vi "DataLogging.vi"(4 "Tab?":bool, 6 "New Line?":bool, 7 "Name":string, 8 "error in (no error)":errorcluster, 10 "WriteToFile?":bool, 11 "Variant In":variant) -> (0 "error out":errorcluster, 3 "FinalText":string)   [LabVIEW 2017]
uses:
  <vilib>/Utility/Data Type/Type Definitions/Data Type.ctl
  <vilib>/Utility/Data Type/NI_Data Type.lvlib
panel:
  out "Type":T1
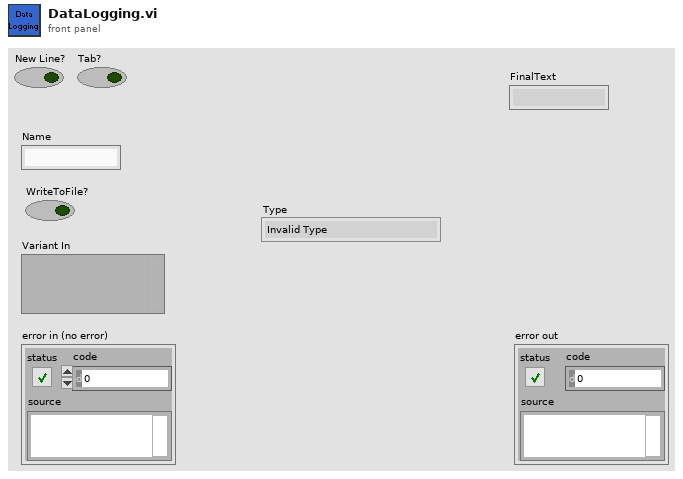
[diagram p1: front panel]
types:
  T1 = typedef "NI_Data Type.lvlib/Data Type.ctl" = enum8{"Invalid Type", "Void", "I8", "I16", "I32", "I64", "U8", "U16", "U32", "U64", "Single Float", "Double Float", "Extended Float", "Single Complex", "Double Complex", "Extended Complex", "Enum U8", "Enum U16", "Enum U32", "Enum U64", "Single Float With Unit", "Double Float With Unit", "Extended Float With Unit", "Single Complex with Unit", "Double Complex with Unit", "Extended Complex with Unit", "Boolean", "String", "Path", "Picture", "Tag", "Array", "Cluster", "Variant", "LV Variant", "Waveform", "Timestamp", "Digital Waveform", "Digital Data", "ExpressData", "Refnum", "External Data", "VI", "Poly VI", "LabVIEW Class Instance", "Fixed Point"}
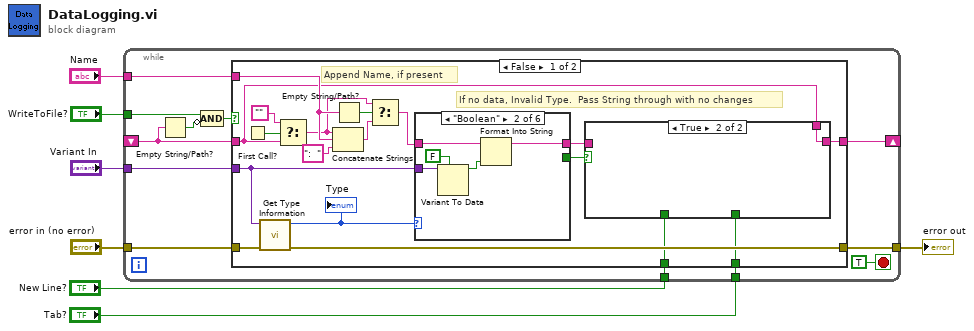
[diagram p0: block diagram]
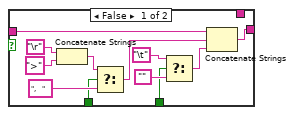
[diagram p2: hidden frame]
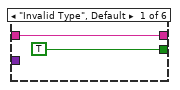
[diagram p3: hidden frame]
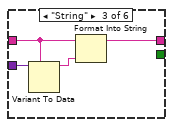
[diagram p4: hidden frame]
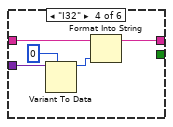
[diagram p5: hidden frame]
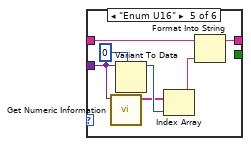
[diagram p6: hidden frame]
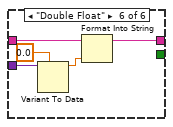
[diagram p7: hidden frame]
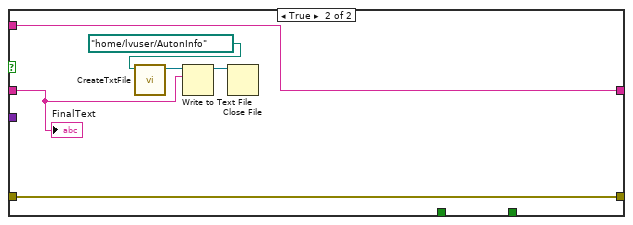
[diagram p8: hidden frame]
diagram:
  n1 = while {
    tunnel: "Variant In" -> [w19]
    shift-right: [w13] -> _
    shift-left: _ -> [w11]
    tunnel: "WriteToFile?" -> [w9]
    tunnel: "error in (no error)" -> [w17]
    tunnel: [w16] -> w4
    tunnel: "Name" -> [w15]
    tunnel: "New Line?" -> [w14]
    tunnel: "Tab?" -> [w12]
    stop <- TRUE stop-if-true
    n2 = Empty String/Path?(string/path=w11) -> (empty?=w8:bool)
    n3 = Compound Arithmetic op=AND(w9, invert w8) -> (w10:bool)
    n4 = case shown="False" w10 {
      tunnel: w19 -> [w37 _]
      tunnel: w17 -> [w36 w84]
      tunnel: [w35 w84] -> w16
      tunnel: w11 -> [w20 w80]
      tunnel: w15 -> [w31 w83]
      tunnel: w14 -> [w26 _]
      tunnel: [w21 w83] -> w13
      tunnel: w12 -> [w24 _]
      frame False {
        # "If no data, Invalid Type.  Pass String through with no changes"
        # "Append Name, if present"
        n5 = First Call?() -> (First Call?: T/F=w33:bool)
        n6 = call <vilib>:"Get Type Information.vi"("error in (no error)"=w36, "Variant"=w37) -> ("error out"=w35:errorcluster, "Type"=w23:T1)  [unwired: 5 in, 3 out]
        "Type" <- w23
        n7 = Select(t="", s=w33, f=w20) -> (s? t:f=w28:string)
        n8 = Concatenate Strings(w28, w31, ":  " ("string")) -> (w29:string)
        n9 = Empty String/Path?(string/path=w31) -> (empty?=w32:bool)
        n10 = Select(t=w28, s=w32, f=w29) -> (s? t:f=w30:string)
        n11 = case shown="\"Boolean\"" w23 {
          tunnel: w37 -> [_ w57 w61 w66 w69 w76]
          tunnel: [w52 w54 w59 w64 w73 w78] -> w25
          tunnel: w30 -> [w52 w53 w58 w63 w72 w77]
          tunnel: [TRUE _ _ _ _ _] -> w22
          frame "Invalid Type", Default {
          }
          frame "Boolean" {
            n12 = Variant To Data(type=FALSE, Variant=w57) -> (data=w55:bool)  [unwired: 1 in, 1 out]
            n13 = Format Into String(initial string=w53, w55) -> (resulting string=w54:string)  [unwired: 2 in, 1 out]
          }
          frame "String" {
            n14 = Variant To Data(type=w58, Variant=w61) -> (data=w60:string)  [unwired: 1 in, 1 out]
            n15 = Format Into String(initial string=w58, w60) -> (resulting string=w59:string)  [unwired: 2 in, 1 out]
          }
          frame "I32" {
            n16 = Variant To Data(type=0, Variant=w66) -> (data=w65:i32)  [unwired: 1 in, 1 out]
            n17 = Format Into String(initial string=w63, w65) -> (resulting string=w64:string)  [unwired: 2 in, 1 out]
          }
          frame "Enum U16" {
            n18 = call <vilib>:"Get Numeric Information.vi"("Variant"=w69) -> ("Enum Names"=w70:string[])  [unwired: 7 in, 3 out]
            n19 = Variant To Data(type=0, Variant=w69) -> (data=w71:i32)  [unwired: 1 in, 1 out]
            n20 = Index Array(array=w70, index=w71) -> (element=w68:string)
            n21 = Format Into String(initial string=w72, w68) -> (resulting string=w73:string)  [unwired: 2 in, 1 out]
          }
          frame "Double Float" {
            n22 = Variant To Data(type=0.0, Variant=w76) -> (data=w74:dbl)  [unwired: 1 in, 1 out]
            n23 = Format Into String(initial string=w77, w74) -> (resulting string=w78:string)  [unwired: 2 in, 1 out]
          }
        }
        n24 = case shown="True" w22 {
          tunnel: w26 -> [w46 _]
          tunnel: w25 -> [w45 _]
          tunnel: w24 -> [w39 _]
          tunnel: [w38 w50] -> w21
          tunnel: w20 -> [_ w50]
          frame False {
            n25 = Concatenate Strings("\r", ">") -> (w47:string)
            n26 = Select(t=w47, s=w46, f=",   ") -> (s? t:f=w44:string)
            n27 = Select(t="\t", s=w39, f="") -> (s? t:f=w42:string)
            n28 = Concatenate Strings(w45, w44, w42) -> (w38:string)
          }
          frame True {
          }
        }
      }
      frame True {
        n29 = call "CreateTxtFile.vi"("pathIn"=path "/home/lvuser/AutonInfo") -> ("refnumOut"=w81:refnum<file>)  [unwired: 10 in]
        n30 = Write to Text File(file (use dialog)=w81, text=w80) -> (refnum out=w82:refnum<file>)  [unwired: 2 in, 2 out]
        n31 = Close File(refnum=w82) -> ()  [unwired: 1 in, 2 out]
        "FinalText" <- w80
      }
    }
  }
  "error out" <- w4
